vi "checkFinishEnemyPossessionAtEnemyFieldPlay.vi"(8 "error in (no error)":errorcluster, 10 "Game":refnum<class "Game.lvclass">, 11 "EnemyPossessionAtEnemyFieldPlay in":refnum<class "EnemyPossessionAtEnemyFieldPlay.lvclass">) -> (0 "error out":errorcluster, 2 "Boolean":bool, 3 "EnemyPossessionAtEnemyFieldPlay out":refnum<class "EnemyPossessionAtEnemyFieldPlay.lvclass">)   [LabVIEW 2018, in "EnemyPossessionAtEnemyFieldPlay.lvclass"]
uses:
  EnemyPossessionAtEnemyFieldPlay.lvclass
  Game_class/Game.lvclass
  Referee_class/command_interpreted.ctl
  Game_class/Game.lvclass/Game.ctl
  Referee_class/Referee.lvclass/Referee.ctl
  Object_class/Object.lvclass/Object.ctl
  Events_class/Events.lvclass/Events.ctl
  Game_class/Read Referee.vi
  Game_class/Read EventsRef.vi
  Game_class/Read BallRef.vi
  Object_class/Read x.vi
  Events_class/Read ball_out.vi
  Events_class/Read enemy_ball_possesion.vi
  Referee_class/Read command_interpreted.vi
  Ball_class/Ball.lvclass
  C:/Users/anton/Desktop/roboime/dar push/SSL_AI/SSL_AI/Object_class/Object.lvclass
  Referee_class/Referee.lvclass
  Events_class/Events.lvclass
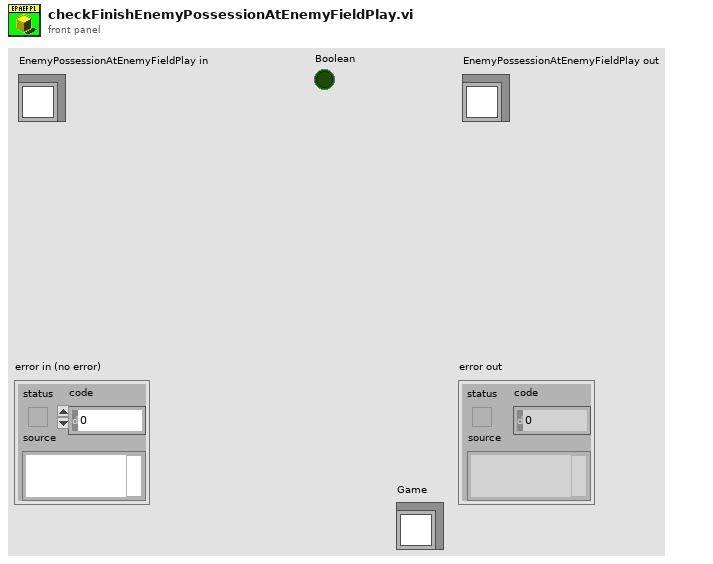
[diagram p1: front panel]
types:
  T1 = typedef "command_interpreted.ctl" = enum16{"Goal Ally", "Goal Enemy", "Ball Placement Enemy", "Ball Placement Ally", "Normal Half Time", "Extra Time  Break", "Extra Half Time", "None", "Post Game", "PKA Normal Start", "Prepare Kickoff Ally", "PKE Normal Start", "Prepare Kickoff Enemy", "Force Start", "Halt", "Timeout", "Prepare Penalty Ally", "Prepare Penalty Enemy", "PPA NormalStart", "PPE Normal Start", "Indirect Free Ally", "Direct Free Enemy", "Direct Free Ally", "Indirect Free Enemy", "Stop"}
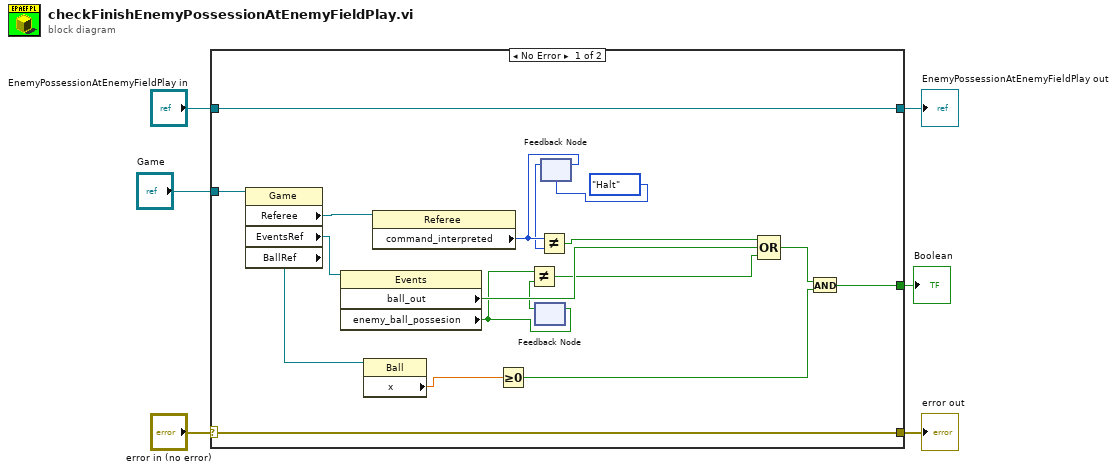
[diagram p0: block diagram]
diagram:
  n1 = case shown="No Error" "error in (no error)" {
    selector: "error in (no error)" -> [w23 w26]
    tunnel: [w23 w26] -> w5
    tunnel: [w24 w25] -> w3
    tunnel: "EnemyPossessionAtEnemyFieldPlay in" -> [w24 w25]
    tunnel: "Game" -> [w18 _]
    tunnel: [w7 _] -> w1
    frame No Error {
      n2 = property class="Game"(reference=w18) -> ("Referee"=w22:refnum<class "Referee.lvclass">, "EventsRef"=w17:refnum<class "Events.lvclass">, "BallRef"=w11:refnum<class "Ball.lvclass">)  [unwired: 1 in, 2 out]
      n3 = property class="Events"(reference=w17) -> ("ball_out"=w15:bool, "enemy_ball_possesion"=w14:bool)  [unwired: 1 in, 2 out]
      n4 = property class="Ball"(reference=w11) -> ("x"=w10:dbl)  [unwired: 1 in, 2 out]
      n5 = property class="Referee"(reference=w22) -> ("command_interpreted"=w21:T1)  [unwired: 1 in, 2 out]
      n6 = Greater Or Equal To 0?(x=w10) -> (x >= 0?=w8:bool)
      n7 = feedback-in #1(w14) -> ()
      n8 = feedback #1() -> (w13:bool)  [unwired: 1 in]
      n9 = Not Equal?(x=w14, y=w13) -> (x != y?=w12:bool)
      n10 = feedback #2(command_interpreted."Halt" ("command_interpreted")) -> (w20:T1)
      n11 = Not Equal?(x=w21, y=w20) -> (x != y?=w16:bool)
      n12 = feedback-in #2(w21) -> ()
      n13 = Compound Arithmetic op=OR(w16, w15, w12) -> (w9:bool)
      n14 = And(x=w9, y=w8) -> (x .and. y?=w7:bool)
    }
    frame Error {
    }
  }
  "error out" <- w5
  "EnemyPossessionAtEnemyFieldPlay out" <- w3
  "Boolean" <- w1
